vi "Update Bus B Pointers.vi"(8 "error in (no error)":errorcluster, 9 "Data Pointers":u16[](array[numeric]), 10 "Command Words":u16[](array[numeric]), 11 "Bus Monitor in":refnum<class "Bus Monitor.lvclass">) -> (0 "error out":errorcluster, 3 "Bus Monitor out":refnum<class "Bus Monitor.lvclass">)   [LabVIEW 2020, in "BCI-1553 API.lvlib" / "Bus Monitor.lvclass"]
doc: "Reads all the Bus B filters and updates their data pointers. If there is still a valid or new data pointer in memory for the filter parameters, they receive that pointer. If there is no command in memory, the parameter data pointer is set to zero. Zero is used as a flag for later to indicate a no change in data."
uses:
  Bus Monitor.lvclass
  Bus Monitor.lvclass/Bus Monitor.ctl
  Dependencies/Registry/Registry.lvclass/Registry.ctl
  Filters/Filter/Filter.lvclass
  Dependencies/Registry/Registry.lvclass
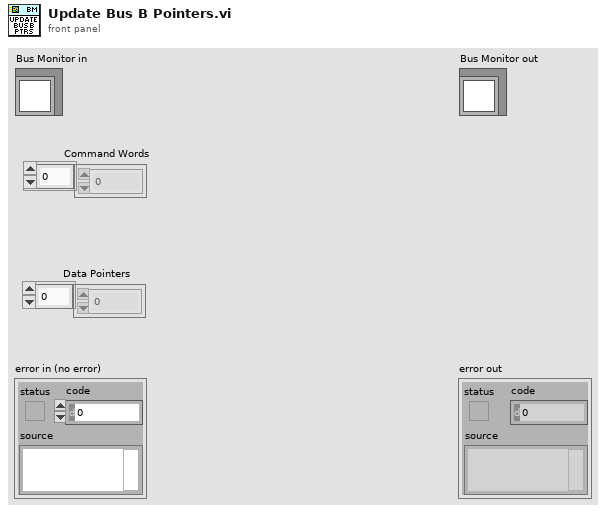
[diagram p1: front panel]
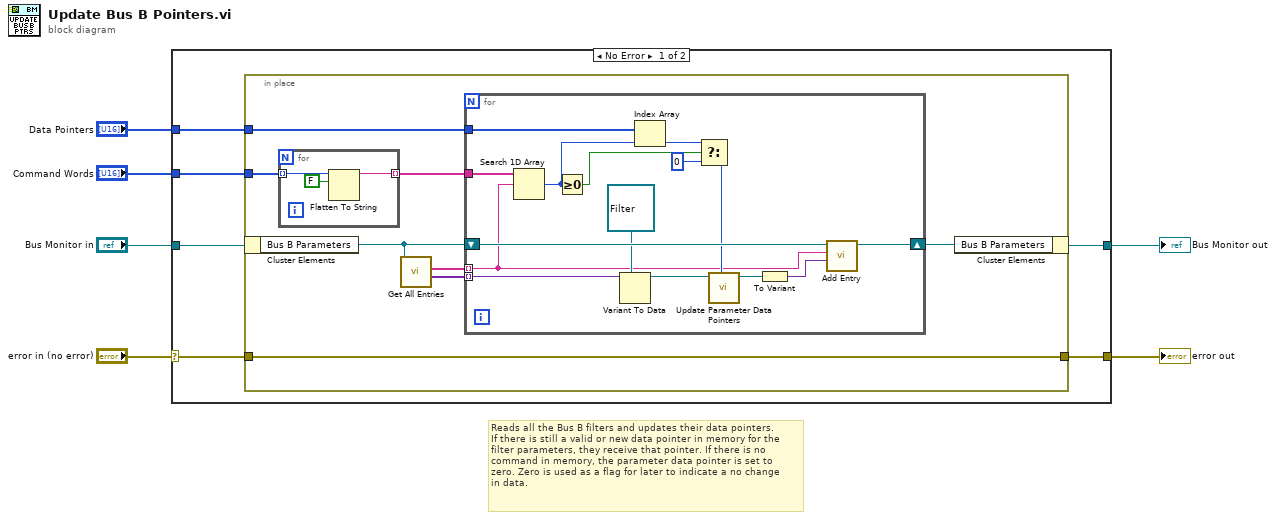
[diagram p0: block diagram]
diagram:
  # "Reads all the Bus B filters and updates their data pointers.\nIf there is still a valid or new data pointer in memory for the\nfilter parameters, they receive that pointer. If there is no\ncommand in memory, the parameter data pointer is set to\nzero. Zero is used as a flag for later to indicate a no change\nin data."
  n1 = case shown="No Error" "error in (no error)" {
    selector: "error in (no error)" -> [w8 w40]
    tunnel: [w9 w40] -> w2
    tunnel: [w10 w39] -> w1
    tunnel: "Bus Monitor in" -> [w7 w39]
    tunnel: "Command Words" -> [w12 _]
    tunnel: "Data Pointers" -> [w11 _]
    frame No Error {
      n2 = in-place {
        in-place-border: w12 -> [w19]
        in-place-border: w11 -> [w13]
        in-place-border: [w20] -> w9
        in-place-border: w8 -> [w20]
        n3 = in-place-cluster #1(w7) -> ("Bus B Parameters"=w16:refnum<class "Registry.lvclass">)
        n4 = for {
          tunnel: w19 -> [w38] mode=indexing
          tunnel: [w36] -> w14 mode=indexing
          n5 = Flatten To String(anything=w38, prepend array or string size? (T)=FALSE) -> (data string=w36:string)  [unwired: 2 in, 2 out]
        }
        n6 = call "Get All Entries.vi"("Registry in"=w16) -> ("Values"=w17:variant[], "Keys"=w18:string[])  [unwired: 8 in, 1 out]
        n7 = for {
          tunnel: w18 -> [w21] mode=indexing
          tunnel: w17 -> [w30] mode=indexing
          shift-right: [w35] -> w15
          shift-left: w16 -> [w34]
          tunnel: w14 -> [w33]
          tunnel: w13 -> [w32]
          n8 = Search 1D Array(1D array=w33, element=w21) -> (index of element=w31:i32)  [unwired: 1 in]
          n9 = Greater Or Equal To 0?(x=w31) -> (x >= 0?=w27:bool)
          n10 = Variant To Data(type=refnum<class "Filter.lvclass"> refnum ("SLSC 1553 API.lvlib:Filter.lvclass"), Variant=w30) -> (data=w28:refnum<class "Filter.lvclass">)  [unwired: 1 in, 1 out]
          n11 = Index Array(array=w32, index=w31) -> (element=w26:u16)
          n12 = Select(t=w26, s=w27, f=u16 0) -> (s? t:f=w24:u16)
          n13 = call-dynamic "Update Parameter Data Pointers.vi"("Data Pointer"=w24, "Filter in"=w28) -> ("Filter out"=w23:refnum<class "Filter.lvclass">)  [unwired: 8 in, 1 out]
          n14 = To Variant(anything=w23) -> (Variant=w22:variant)
          n15 = call "Add Entry.vi"("Value"=w22, "Key"=w21, "Registry in"=w34) -> ("Registry out"=w35:refnum<class "Registry.lvclass">)  [unwired: 6 in, 2 out]
        }
        n16 = in-place-cluster #1("Bus B Parameters"=w15) -> (w10:refnum<class "Bus Monitor.lvclass">)
      }
    }
    frame Error {
    }
  }
  "error out" <- w2
  "Bus Monitor out" <- w1
